vi "ocr unit.vi"(6 "File Path in":path, 8 "image features":T2, 9 "select source":enum32{"user selectable", "constant"}(ring), 10 "reject roi border particles":bool, 11 "Refnum in":T1) -> (0 "angle of rotation":dbl, 1 "Array":string[](array[string]), 2 "Read String":string, 3 "Refnum out":T1, 4 "image rotated by :":dbl)   [LabVIEW 2011]
uses:
  <vilib>/vision/Image Controls.llb/IMAQ Image.ctl
  <vilib>/vision/NI_Vision_Development_Module.lvlib
panel:
  out "Image":T1(plugin-control)
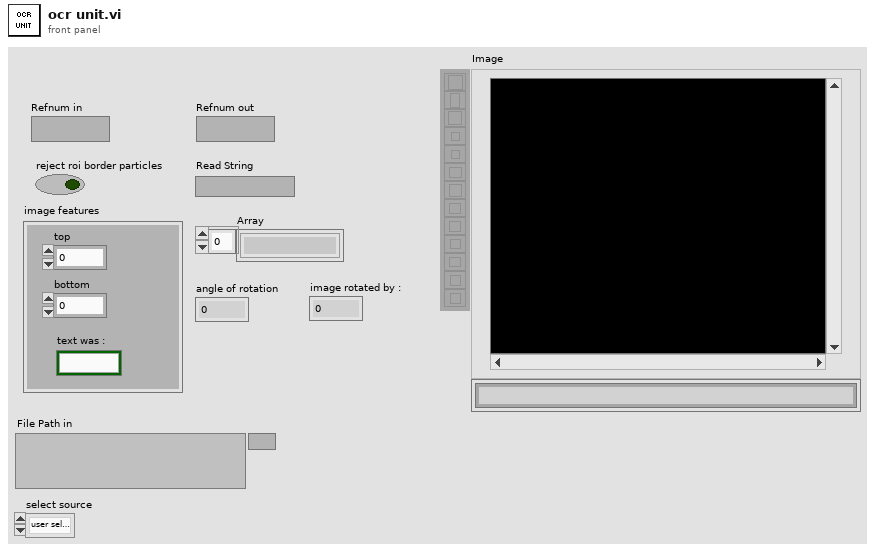
[diagram p1: front panel]
types:
  T1 = typedef "IMAQ Image.ctl" = refnum<image>
  T2 = cluster{"text was :":bool, "top":i32, "bottom":i32}
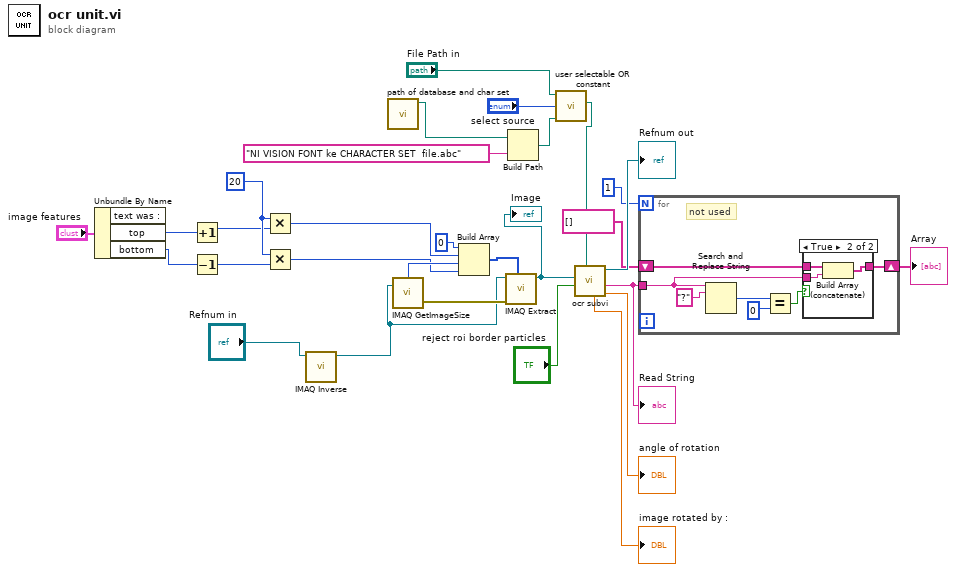
[diagram p0: block diagram]
diagram:
  w10 = 20 ("y")
  n1 = Unbundle By Name("image features") -> ("top"=w13:i32, "bottom"=w12:i32)  [unwired: 1 out]
  n2 = Increment(x=w13) -> (x+1=w9:i32)
  n3 = Decrement(x=w12) -> (x-1=w8:i32)
  n4 = Multiply(x=w10, y=w9) -> (x*y=w16:i32)
  n5 = Multiply(x=w10, y=w8) -> (x*y=w11:i32)
  n6 = call "IMAQ Inverse"("Image Src"="Refnum in") -> ("Image Dst Out"=w6:T1)  [unwired: 9 in, 1 out]
  n7 = call "path of database and char set.vi"() -> ("appended path"=w22:path)  [unwired: 11 in]
  n8 = call "IMAQ GetImageSize"("Image"=w6) -> ("X Resolution"=w15:i32, "error out"=w17:errorcluster)  [unwired: 3 in, 1 out]
  n9 = Build Array(0, w16, w15, w11) -> (w19:i32[])
  n10 = call "IMAQ Extract"("Optional Rectangle"=w19, "error in (no error)"=w17, "Image Src"=w6) -> ("Image Dst Out"=w5:T1)  [unwired: 7 in, 1 out]
  "Image" <- w5
  n11 = Build Path(base path=w22, name or relative path="NI VISION FONT ke CHARACTER SET  file.abc") -> (appended path=w3:path)
  n12 = call "user selectable OR constant.vi"("Constant Path in"=w3, "select source"="select source", "File Path in"="File Path in") -> ("appended path"=w4:path)  [unwired: 8 in]
  n13 = call "ocr subvi.vi"("char set file path"=w4, "reject roi border particles"="reject roi border particles", "Image"=w5) -> ("calc angle of rotation"=→"angle of rotation":dbl, "Read String"=w24:string, "Image 2"=→"Refnum out":T1, "image rotated by :"=→"image rotated by :":dbl)  [unwired: 5 in]
  "Read String" <- w24
  n14 = for {
    N: 1 -> [_]
    tunnel: w24 -> [w34]
    shift-right: [w36] -> w25
    shift-left: string[] [] -> [w35]
    # "not used"
    n15 = Search and Replace String(input string=w34, search string="?" ("string")) -> (number of replacements=w32:i32)  [unwired: 6 in, 3 out]
    n16 = Equal?(x=w32, y=0) -> (x = y?=w30:bool)
    n17 = case shown="True" w30 {
      tunnel: w34 -> [_ w40]
      tunnel: [w37 w39] -> w36
      tunnel: w35 -> [w37 w38]
      frame False {
      }
      frame True {
        n18 = Build Array (concatenate)(w38, w40) -> (w39:string[])
      }
    }
  }
  "Array" <- w25
